vi "Get_Image_File_Paths_from_AD_Dataset.vi"(6 "Good Folder Names":string[](array[string])=["good", "Good"], 8 "error in":errorcluster, 11 "Dataset Folder":path) -> (0 "error out":errorcluster, 2 "Bad Dataset Files":path[](array[path]), 3 "Good Dataset Files":path[](array[path]))   [LabVIEW 2024]
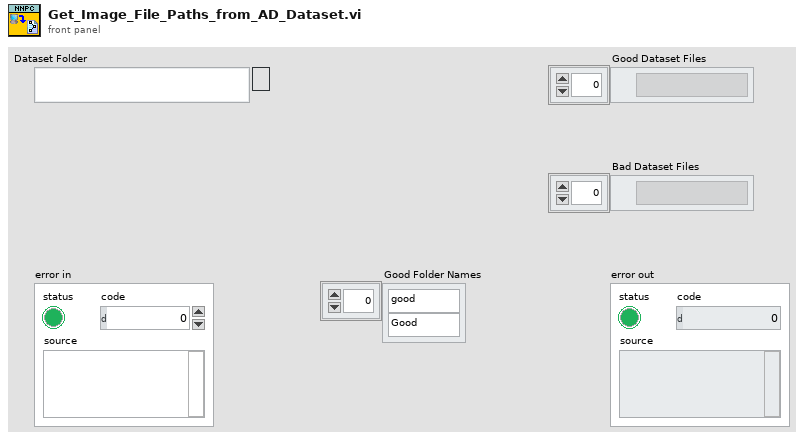
[diagram p1: front panel]
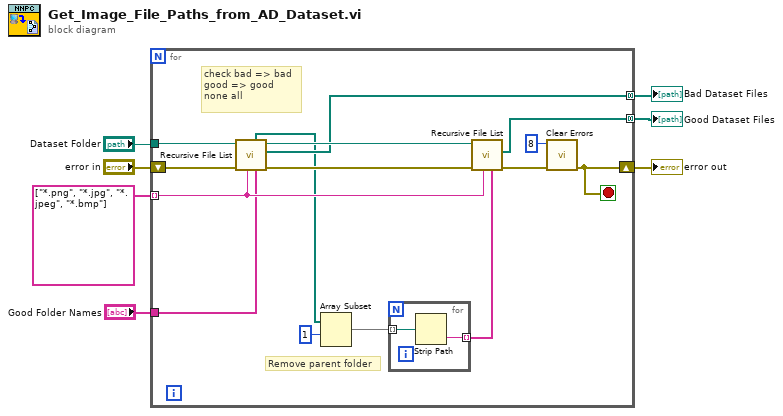
[diagram p0: block diagram]
diagram:
  n1 = for {
    tunnel: "Dataset Folder" -> [w15]
    tunnel: string[] ["*.png", "*.jpg", "*.jpeg", "*.bmp"] ("pattern") -> [w14] mode=indexing
    tunnel: [w17] -> w2 mode=concatenating
    tunnel: [w16] -> w1 mode=concatenating
    tunnel: "Good Folder Names" -> [w12]
    shift-right: [w8] -> w6
    shift-left: "error in" -> [w13]
    stop <- w8 stop-if-true
    # "Remove parent folder"
    # "check bad => bad\ngood => good\nnone all"
    n2 = call <vilib>:"Recursive File List.vi"("Folders to Exclude"=w12, "pattern"=w14, "error in (no error)"=w13, "Folder Path"=w15) -> ("error out"=w19:errorcluster, "All Files in Dir"=w17:path[], "dup Folder Path"=w21:path, "All Folders"=w11:path[])  [unwired: 3 in, 1 out]
    n3 = Array Subset(array=w11, index=1) -> (w10:path[])  [unwired: 1 in]
    n4 = for {
      tunnel: w10 -> [w24] mode=indexing
      tunnel: [w23] -> w9 mode=indexing
      n5 = Strip Path(path=w24) -> (name=w23:string)  [unwired: 1 out]
    }
    n6 = call <vilib>:"Recursive File List.vi"("Folders to Exclude"=w9, "pattern"=w14, "error in (no error)"=w19, "Folder Path"=w21) -> ("error out"=w18:errorcluster, "All Files in Dir"=w16:path[])  [unwired: 3 in, 3 out]
    n7 = call <vilib>:"Clear Errors.vi"("error in (no error)"=w18, "specific error code to clear (0: all)"=8) -> ("error out"=w8:errorcluster)  [unwired: 4 in, 1 out]
  }
  "error out" <- w6
  "Good Dataset Files" <- w1
  "Bad Dataset Files" <- w2
